vi "RPLiDAR_S2_Parser_KBS_실습용.vi"() -> ()   [LabVIEW 2023]
uses:
  20aa278b-1264-4e69-9e98-0b58d0a71f5b.vi
  <vilib>/Instr/_visa.llb/VISA Configure Serial Port (Instr).vi
panel:
  in  "Tab Control":T1(tab)
  in  "COM4":refnum<visa-resource-name>="COM29" caption="S2_PORT"
  out "Loop Time":u32=100
  out "read buffer":string
  out "RAW DATA SIZE":i32
  out "RAW XY":cluster{dbl[], "Y":dbl[]}(graph)
  out "XY IN ROI":cluster{dbl[], "Y":dbl[]}[](graph)=[{[3000.0, 3000.0, -3000.0, -3000.0, 3000.0], "Y"=[-1000.0, 3000.0, 3000.0, -1000.0, -1000.0]}, {[], "Y"=[]}]
  in  "X+ limit":dbl=3000.0
  in  "X- limit":dbl=-3000.0
  in  "Y+ limit":dbl=3000.0
  in  "Y- limit":dbl=-1000.0
  out "XY IN ROI DATA SIZE":i32
  out "XY GRID":cluster{i32[], i32[]}(graph)
  in  "GRID Filter":i32=1
  out "GRIDED XY DATA SIZE":i32
  out "CLUSTERD XY":cluster{i32[], i32[]}[](graph)
  in  "MIN SIZE":i32=10
  in  "MAX SIZE":i32=300
  in  "유클리디언":dbl=200.0
  in  "stop":bool
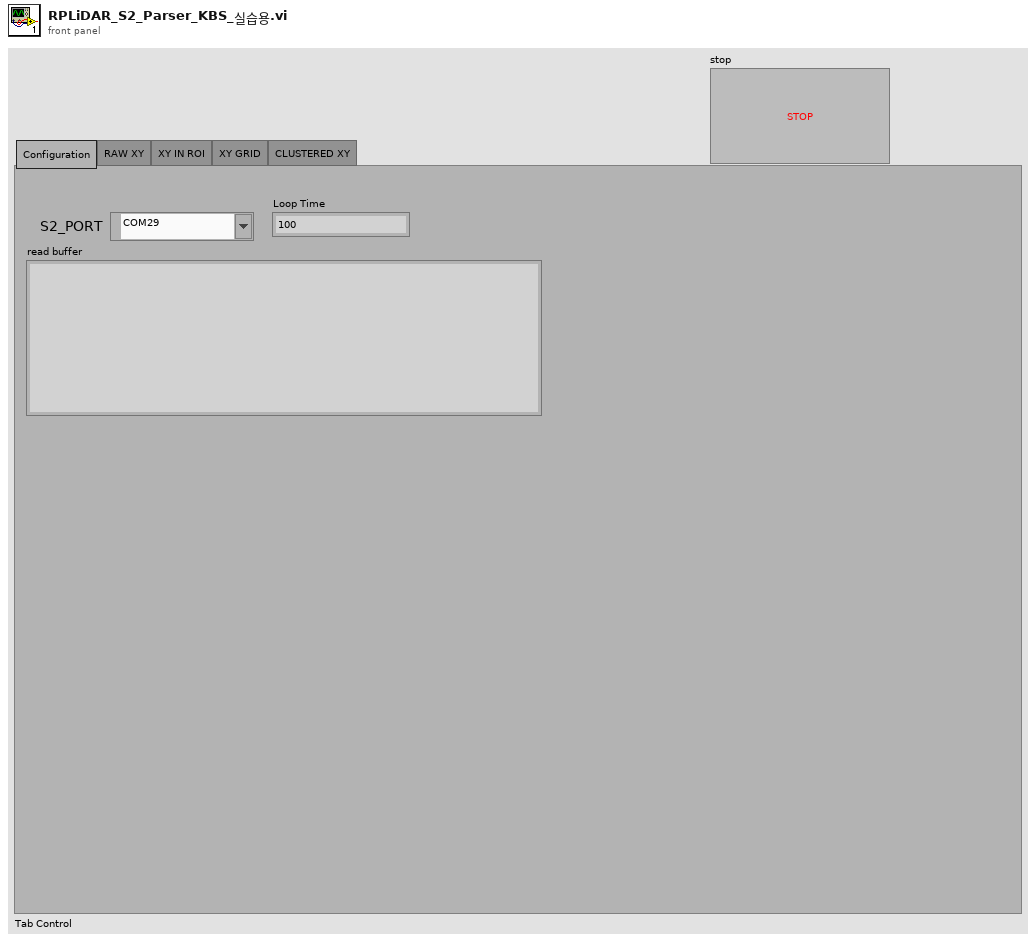
[diagram p1: front panel]
types:
  T1 = enum32{"Configuration", "RAW XY", "XY IN ROI", "XY GRID", "CLUSTERED XY"}
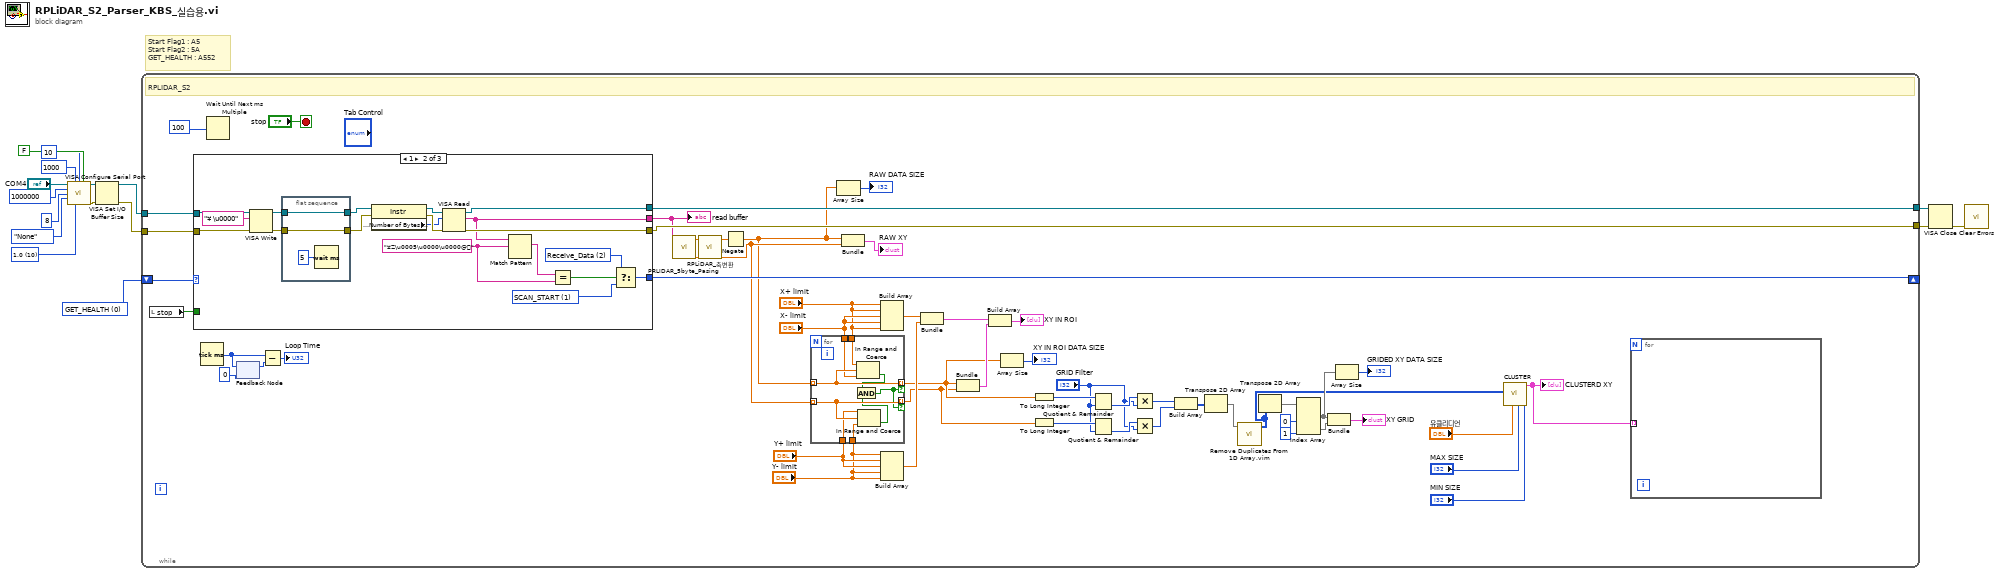
[diagram p0: block diagram]
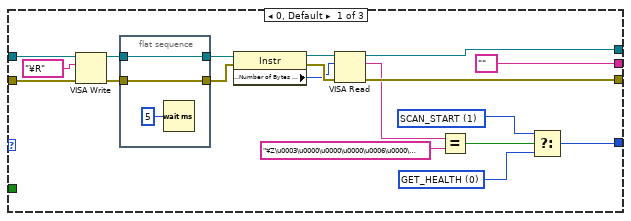
[diagram p2: hidden frame]
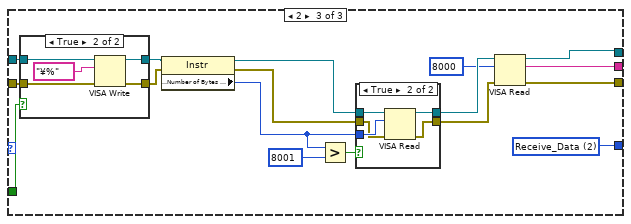
[diagram p3: hidden frame]
diagram:
  w1 = u16 10 items=["1.0"=10, "1.5"=15, "2.0"=20] ("stop bits (10: 1 bit)")
  w3 = u16 0 items=["GET_HEALTH", "SCAN_START", "Receive_Data"]
  # "Start Flag1 : A5\nStart Flag2 : 5A \nGET_HEALTH : A552"
  n1 = call-poly "VISA Configure Serial Port"("VISA resource name"="COM4", "timeout (10sec)"=u32 1000, "termination char\n(0xA = '\\n' = LF)"=u8 10 ("termination char\n(0xA = '\\n' = LF)"), "Enable Termination\nChar (T)"=FALSE ("Enable Termination\nChar (T)"), "baud rate (9600)"=u32 1000000, "data bits (8)"=u16 8, "parity (0:none)"=enum16{"None", "Odd", "Even", "Mark", "Space"}."None", "stop bits (10: 1 bit)"=w1) -> ("VISA resource name out"=w11:refnum<visa-resource-name>, "error out"=w10:errorcluster)  [unwired: 6 in]
  n2 = VISA Set I/O Buffer Size(VISA resource name=w11, error in (no error)=w10) -> (VISA resource name out=w5:refnum<visa-resource-name>, error out=w4:errorcluster)  [unwired: 2 in]
  n3 = while {
    tunnel: [w59] -> w15
    tunnel: [w60] -> w14
    tunnel: w5 -> [w68]
    tunnel: w4 -> [w67]
    shift-right: [w66] -> _
    shift-left: w3 -> [w69]
    stop <- "stop" stop-if-true
    # "RPLIDAR_S2"
    n4 = local read "stop"() -> (w65:bool)
    n5 = case shown="1" w69 {
      tunnel: w68 -> [w97 w115 w138]
      tunnel: w67 -> [w96 w114 w137]
      tunnel: [w98 w111 w124] -> w66
      tunnel: [w87 w112 w140] -> w60
      tunnel: [w86 w113 w139] -> w59
      tunnel: w65 -> [_ _ w136]
      tunnel: ["" ("read buffer") w109 w135] -> w55
      frame 0, Default {
        w80 = u16 0 items=["GET_HEALTH", "SCAN_START", "Receive_Data"]
        w81 = u16 1 items=["GET_HEALTH", "SCAN_START", "Receive_Data"]
        n6 = VISA Write(VISA resource name=w97, write buffer="¥R", error in (no error)=w96) -> (VISA resource name out=w91:refnum<visa-resource-name>, error out=w90:errorcluster)  [unwired: 1 out]
        n7 = flat-sequence {
          tunnel: w91 -> [w101]
          tunnel: w90 -> [w100]
          tunnel: [w101] -> w89
          tunnel: [w100] -> w88
          frame #0 {
            n8 = Wait (ms)(milliseconds to wait=u32 5 ("대기 시간 (ms)")) -> ()  [unwired: 1 out]
          }
        }
        n9 = property class="Instr"(reference=w89, error in=w88) -> (reference out=w94:refnum<visa-resource-name>, error out=w93:errorcluster, "Serial Settings:Number of Bytes at Serial Port"=w92:u32)
        n10 = VISA Read(VISA resource name=w94, byte count=w92, error in (no error)=w93) -> (VISA resource name out=w86:refnum<visa-resource-name>, read buffer=w83:string, error out=w87:errorcluster)  [unwired: 1 out]
        n11 = Equal?(x=w83, y="¥Z\u0003\u0000\u0000\u0000\u0006\u0000\u0000\u0000") -> (x = y?=w84:bool)
        n12 = Select(t=w81, s=w84, f=w80) -> (s? t:f=w98:u16)
      }
      frame 1 {
        w102 = u16 2 items=["GET_HEALTH", "SCAN_START", "Receive_Data"]
        w103 = u16 1 items=["GET_HEALTH", "SCAN_START", "Receive_Data"]
        w116 = "¥Z\u0005\u0000\u0000@"
        n13 = VISA Write(VISA resource name=w115, write buffer="¥ \u0000", error in (no error)=w114) -> (VISA resource name out=w118:refnum<visa-resource-name>, error out=w119:errorcluster)  [unwired: 1 out]
        n14 = flat-sequence {
          tunnel: w118 -> [w123]
          tunnel: w119 -> [w122]
          tunnel: [w123] -> w105
          tunnel: [w122] -> w104
          frame #0 {
            n15 = Wait (ms)(milliseconds to wait=u32 5 ("대기 시간 (ms)")) -> ()  [unwired: 1 out]
          }
        }
        n16 = property class="Instr"(reference=w105, error in=w104) -> (reference out=w108:refnum<visa-resource-name>, error out=w107:errorcluster, "Serial Settings:Number of Bytes at Serial Port"=w106:u32)
        n17 = VISA Read(VISA resource name=w108, byte count=w106, error in (no error)=w107) -> (VISA resource name out=w113:refnum<visa-resource-name>, read buffer=w109:string, error out=w112:errorcluster)  [unwired: 1 out]
        n18 = Match Pattern(string=w109, regular expression=w116) -> (match substring=w110:string)  [unwired: 1 in, 3 out]
        n19 = Equal?(x=w110, y=w116) -> (x = y?=w120:bool)
        n20 = Select(t=w102, s=w120, f=w103) -> (s? t:f=w111:u16)
      }
      frame 2 {
        w124 = u16 2 items=["GET_HEALTH", "SCAN_START", "Receive_Data"]
        n21 = case shown="True" w136 {
          tunnel: w138 -> [w149 w153]
          tunnel: w137 -> [w148 w152]
          tunnel: [w149 w151] -> w134
          tunnel: [w148 w150] -> w133
          frame False {
          }
          frame True {
            n22 = VISA Write(VISA resource name=w153, write buffer="¥%", error in (no error)=w152) -> (VISA resource name out=w151:refnum<visa-resource-name>, error out=w150:errorcluster)  [unwired: 1 out]
          }
        }
        n23 = property class="Instr"(reference=w134, error in=w133) -> (reference out=w129:refnum<visa-resource-name>, error out=w128:errorcluster, "Serial Settings:Number of Bytes at Serial Port"=w130:u32)
        n24 = Greater?(x=w130, y=u32 8001) -> (0:w132:bool)
        n25 = case shown="True" w132 {
          tunnel: w129 -> [w142 w147]
          tunnel: w130 -> [_ w146]
          tunnel: w128 -> [w141 w145]
          tunnel: [w142 w144] -> w127
          tunnel: [w141 w143] -> w126
          frame False {
          }
          frame True {
            n26 = VISA Read(VISA resource name=w147, byte count=w146, error in (no error)=w145) -> (VISA resource name out=w144:refnum<visa-resource-name>, error out=w143:errorcluster)  [unwired: 2 out]
          }
        }
        n27 = VISA Read(VISA resource name=w127, byte count=u32 8000, error in (no error)=w126) -> (VISA resource name out=w139:refnum<visa-resource-name>, read buffer=w135:string, error out=w140:errorcluster)  [unwired: 1 out]
      }
    }
    "read buffer" <- w55
    n28 = Tick Count (ms)() -> (millisecond timer value=w64:u32)
    n29 = Wait Until Next ms Multiple(millisecond multiple=u32 100 ("ms 배수")) -> ()  [unwired: 1 out]
    n30 = feedback #1(u32 0 ("millisecond timer value")) -> (w63:u32)
    n31 = feedback-in #1(w64) -> ()
    n32 = Subtract(x=w64, y=w63) -> (x-y=→"Loop Time":u32)
    n33 = call "PRLIDAR_5byte_Pasing.vi"("RPLIDAR_Data"=w55) -> ("Distance(mm)"=w56:dbl[], "Theta(deg)"=w57:dbl[])  [unwired: 9 in]
    n34 = call "RPLiDAR_축변환.vi"("Distance(mm)"=w56, "Theta(deg)"=w57) -> ("Y"=w50:dbl[], "X"=w51:dbl[])  [unwired: 8 in]
    n35 = Negate(x=w51) -> (-x=w49:dbl[])
    n36 = for {
      tunnel: w49 -> [w79] mode=indexing
      tunnel: w50 -> [w78] mode=indexing
      tunnel: [w79] -> w36 mode=indexing if=w71
      tunnel: [w78] -> w35 mode=indexing if=w71
      tunnel: "X+ limit" -> [w77]
      tunnel: "X- limit" -> [w76]
      tunnel: "Y+ limit" -> [w75]
      tunnel: "Y- limit" -> [w74]
      n37 = In Range and Coerce(upper limit=w77, x=w79, lower limit=w76) -> (In Range?=w73:bool)  [unwired: 1 out]
      n38 = In Range and Coerce(upper limit=w75, x=w78, lower limit=w74) -> (In Range?=w72:bool)  [unwired: 1 out]
      n39 = And(x=w73, y=w72) -> (x .and. y?=w71:bool)
    }
    n40 = Array Size(array=w49) -> (size(s)=→"RAW DATA SIZE":i32)
    n41 = Bundle(w49, "Y"=w50) -> (→"RAW XY":cluster{dbl[], "Y":dbl[]})  [unwired: 1 in]
    n42 = Build Array("X+ limit", "X+ limit", "X- limit", "X- limit", "X+ limit") -> (w42:dbl[])
    n43 = Build Array("Y- limit", "Y+ limit", "Y+ limit", "Y- limit", "Y- limit") -> (w41:dbl[])
    n44 = Bundle(w42, w41) -> (w40:cluster{dbl[], dbl[]})  [unwired: 1 in]
    n45 = Bundle(w36, w35) -> (w39:cluster{dbl[], dbl[]})  [unwired: 1 in]
    n46 = Build Array(w40, w39) -> (→"XY IN ROI":cluster{dbl[], dbl[]}[])
    n47 = Array Size(array=w36) -> (size(s)=→"XY IN ROI DATA SIZE":i32)
    n48 = To Long Integer(number=w36) -> (32bit integer=w34:i32[])
    n49 = To Long Integer(number=w35) -> (32bit integer=w33:i32[])
    n50 = Quotient & Remainder(x=w34, y="GRID Filter") -> (floor(x/y)=w32:i32[])  [unwired: 1 out]
    n51 = Quotient & Remainder(x=w33, y="GRID Filter") -> (floor(x/y)=w31:i32[])  [unwired: 1 out]
    n52 = Multiply(x=w32, y="GRID Filter") -> (x*y=w30:i32[])
    n53 = Multiply(x=w31, y="GRID Filter") -> (x*y=w29:i32[])
    n54 = Build Array(w30, w29) -> (w28:i32[][])
    n55 = Transpose 2D Array(2D array=w28) -> (transposed array=w27:i32[][])
    n56 = call "Remove Duplicates From 1D Array.vim"("array"=w27) -> ("array with duplicates removed"=w18:i32[][])  [unwired: 10 in]
    n57 = Transpose 2D Array(2D array=w18) -> (transposed array=w26:i32[][])
    n58 = Index Array(array=w26, index (row) #1=0 ("index (row)"), index (row) #2=1 ("index (row)")) -> (element #1=w21:i32[], element #2=w23:i32[])  [unwired: 2 in]
    n59 = Bundle(w21, w23) -> (→"XY GRID":cluster{i32[], i32[]})  [unwired: 1 in]
    n60 = Array Size(array=w21) -> (size(s)=→"GRIDED XY DATA SIZE":i32)
    n61 = call "CLUSTER.vi"("MIN SIZE"="MIN SIZE", "MAX SIZE"="MAX SIZE", "유클리디언"="유클리디언", "array with duplicates removed"=w18) -> ("Array"=w17:cluster{i32[], i32[]}[])  [unwired: 7 in]
    "CLUSTERD XY" <- w17
    n62 = for {
      tunnel: w17 -> [_] mode=indexing
    }
  }
  n63 = VISA Close(VISA resource name=w15, error in (no error)=w14) -> (error out=w16:errorcluster)
  n64 = call <vilib>:"Clear Errors.vi"("error in (no error)"=w16) -> ()  [unwired: 5 in, 2 out]
